vi "Benchmark SV Send  LV2012 - NI Verified - 3.vi"() -> ()   [LabVIEW 2015]
panel:
  out "appended array":dbl[](array[numeric])
  in  "Status":string[](array[string])=["Close", "Close", "Close", "Close", "Close", "Close", "Close", "Close"]
  in  "Brake Voltage FB":bool[](array[boolean])=[FALSE, FALSE, FALSE, FALSE, FALSE, TRUE, TRUE, TRUE]
  in  "Motor Voltage FB":bool[](array[boolean])=[FALSE, FALSE, FALSE, FALSE, FALSE, FALSE, FALSE, TRUE]
  in  "Brake":bool[](array[boolean])=[FALSE, FALSE, FALSE, FALSE, FALSE, FALSE, FALSE, TRUE]
  in  "Direction":bool[](array[boolean])=[FALSE, FALSE, FALSE, FALSE, FALSE, FALSE, FALSE, TRUE]
  in  "Enable":bool[](array[boolean])=[FALSE, FALSE, FALSE, FALSE, FALSE, FALSE, FALSE, TRUE]
  in  "Reset":bool
  out "Tries":u32
  out "Average Delay (ms)":dbl
  out "Delay (ms)":u32
  in  "stop":bool
  # "Overview:  Coding that exemplifies how to benchmark the communication of Shared Variables.\nRequirements: LabVIEW 2012 or compatible\nInstructions:\n1.  Run the \"Benchmark SV Receive LV2012 - NI Verified.vi\"\n2. Run this VI\n3. Watch the amount of time it takes to communicate\n4. Stop both VIs"
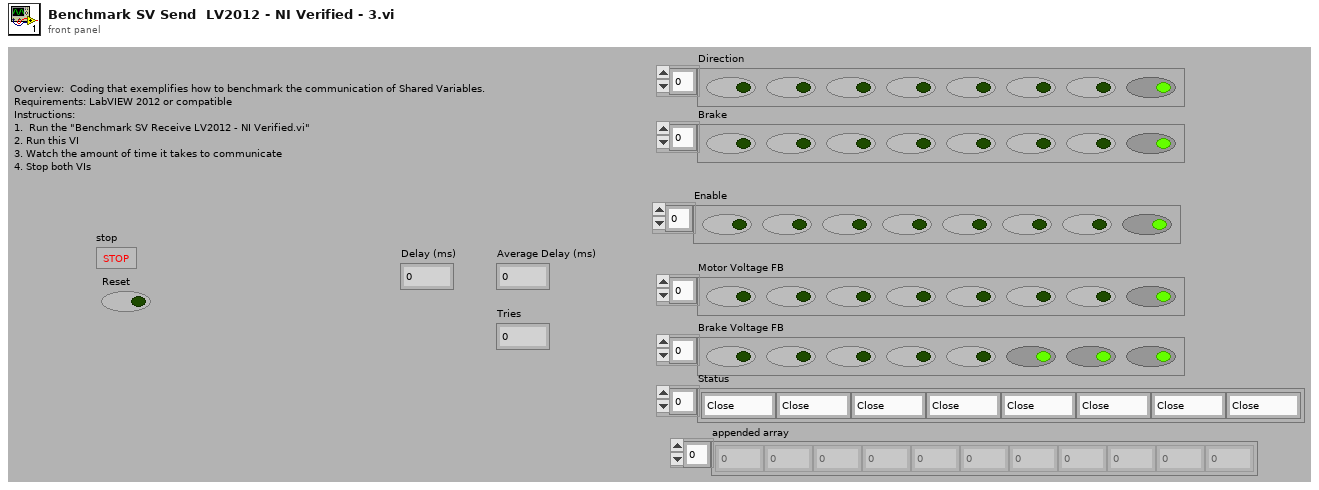
[diagram p1: front panel]
types:
  T1 = cluster{"Built-In Encoder":i32[], "ID":i16[], "Enable":bool[], "Direction":bool[], "Brake":bool[], "Motor Voltage FB":bool[], "Motor Current FB":i32[], "Brake Voltage FB":bool[], "Brake Current FB":i32[], "Status":string[]}
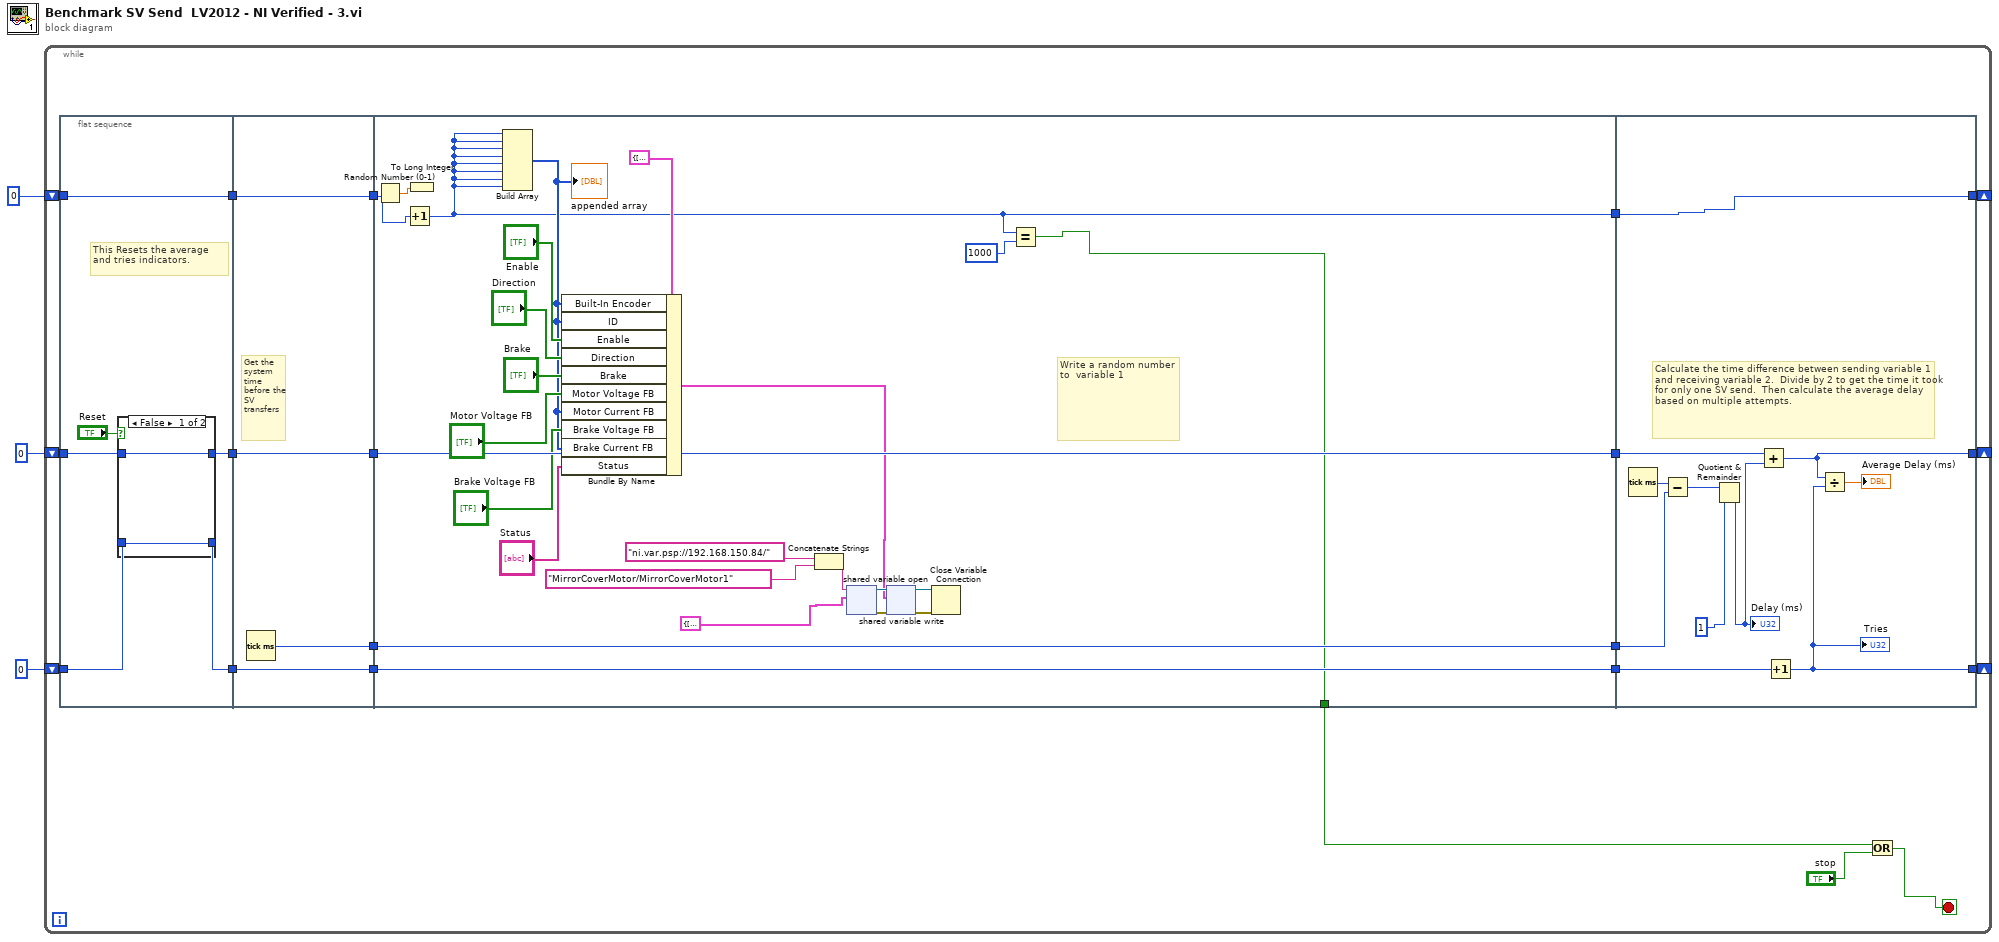
[diagram p0: block diagram]
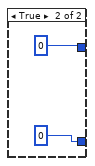
[diagram p2: hidden frame]
diagram:
  n1 = while {
    shift-right: [w22] -> _
    shift-left: u32 0 -> [w12]
    shift-right: [w20] -> _
    shift-left: u32 0 -> [w13]
    shift-right: [w7] -> _
    shift-left: u32 0 -> [w9]
    stop <- w6 stop-if-true
    n2 = flat-sequence {
      tunnel: w12 -> [w29]
      tunnel: [w28] -> w17
      tunnel: [w26] -> w15
      tunnel: w13 -> [w25]
      tunnel: [w24] -> w10
      tunnel: w9 -> [w24]
      tunnel: [w35] -> w18
      tunnel: w17 -> [w37]
      tunnel: [w37] -> w16
      tunnel: w15 -> [w36]
      tunnel: [w36] -> w14
      tunnel: [w34] -> w11
      tunnel: w10 -> [w34]
      tunnel: [w62] -> w23
      tunnel: [w61] -> w21
      tunnel: [w60] -> w19
      tunnel: [w39] -> w8
      tunnel: w11 -> [w41]
      tunnel: w14 -> [w60]
      tunnel: w16 -> [w61]
      tunnel: w18 -> [w62]
      tunnel: [w38] -> w4
      tunnel: w23 -> [w72]
      tunnel: [w65] -> w22
      tunnel: w21 -> [w67]
      tunnel: [w64] -> w20
      tunnel: w19 -> [w71]
      tunnel: w8 -> [w63]
      tunnel: [w63] -> w7
      frame #0 {
        # "This Resets the average \nand tries indicators."
        n3 = case shown="False" "Reset" {
          tunnel: [w31 u32 0] -> w28
          tunnel: w29 -> [w31 _]
          tunnel: [w30 u32 0] -> w26
          tunnel: w25 -> [w30 _]
          frame False {
          }
          frame True {
          }
        }
      }
      frame #1 {
        # "Get the system time before the SV transfers"
        n4 = Tick Count (ms)() -> (millisecond timer value=w35:u32)
      }
      frame #2 {
        # "Write a random number to  variable 1"
        n5 = Random Number (0-1)() -> (number: 0 to 1=w42:dbl)
        n6 = Increment(x=w41) -> (x+1=w39:u32)
        n7 = To Long Integer(number=w42) -> ()  [unwired: 1 out]
        n8 = Build Array(w39, w39, w39, w39, w39, w39, w39, w39) -> (w47:u32[])
        "appended array" <- w47
        n9 = Bundle By Name(cluster=T1 {"Built-In Encoder"=[], "ID"=[], "Enable"=[], "Direction"=[], "Brake"=[], "Motor Voltage FB"=[], "Motor Current FB"=[], "Brake Voltage FB"=[], "Brake Current FB"=[], "Status"=[]} ("input cluster"), "Built-In Encoder"=w47, "ID"=w47, "Enable"="Enable", "Direction"="Direction", "Brake"="Brake", "Motor Voltage FB"="Motor Voltage FB", "Motor Current FB"=w47, "Brake Voltage FB"="Brake Voltage FB", "Brake Current FB"=w47, "Status"="Status") -> (w43:T1)
        n10 = Concatenate Strings("ni.var.psp://192.168.150.84/" ("string"), "MirrorCoverMotor/MirrorCoverMotor1") -> (w55:string)
        n11 = shared-variable-open(w55, T1 {"Built-In Encoder"=[], "ID"=[], "Enable"=[], "Direction"=[], "Brake"=[], "Motor Voltage FB"=[], "Motor Current FB"=[], "Brake Voltage FB"=[], "Brake Current FB"=[], "Status"=[]} ("MirrorCoverMotor")) -> (w59:refnum<k21>, w56:errorcluster)  [unwired: 2 in]
        n12 = shared-variable-write(w59, w56, w43) -> (w57:refnum<k21>, w58:errorcluster)
        n13 = Close Variable Connection(8:w58, 11:w57) -> ()  [unwired: 1 out]
        n14 = Equal?(x=w39, y=1000) -> (x = y?=w38:bool)
      }
      frame #3 {
        # "Calculate the time difference between sending variable 1 and receiving variable 2.  Divide by 2 to get the time it took for only one SV send.  Then calculate the average delay based on multiple attempts."
        n15 = Tick Count (ms)() -> (millisecond timer value=w73:u32)
        n16 = Subtract(x=w73, y=w72) -> (x-y=w70:u32)
        n17 = Quotient & Remainder(x=w70, y=u32 1) -> (floor(x/y)=w68:u32)  [unwired: 1 out]
        "Delay (ms)" <- w68
        n18 = Add(x=w67, y=w68) -> (x+y=w65:u32)
        n19 = Increment(x=w71) -> (x+1=w64:u32)
        "Tries" <- w64
        n20 = Divide(x=w65, y=w64) -> (x/y=→"Average Delay (ms)":dbl)
      }
    }
    n21 = Or(x=w4, y="stop") -> (x .or. y?=w6:bool)
  }
